vi "ClsSignalIdMakerControl.vi"(11 "SignalIDSettings":T1) -> (3 "Array":i32[](array[numeric]))   [LabVIEW 2015]
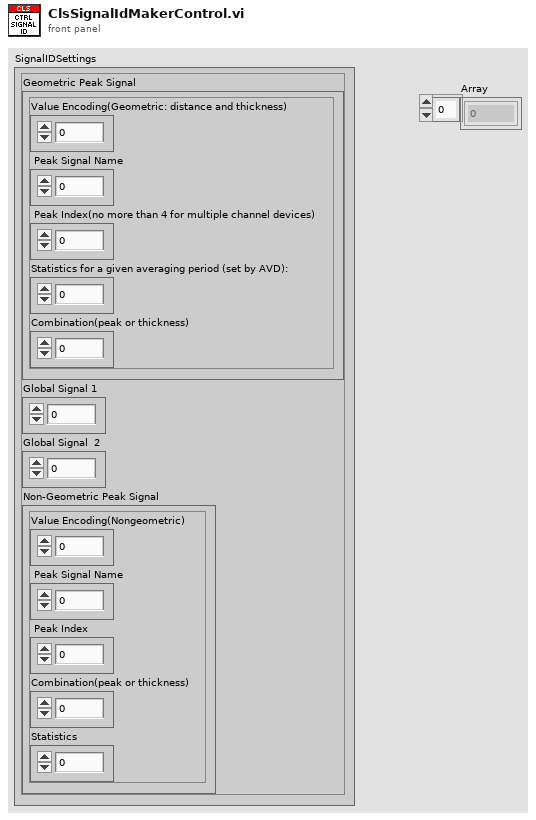
[diagram p1: front panel]
types:
  T1 = cluster{"Geometric Peak Signal":cluster{"Value Encoding(Geometric: distance and thickness) ":i32, " Peak Signal Name":i32, " Peak Index(no more than 4 for multiple channel devices)":i32, "Statistics for a given averaging period (set by AVD):":i32, "Combination(peak or thickness)":i32}, "Global Signal 1":i32, "Global Signal  2":i32, "Non-Geometric Peak Signal":cluster{"Value Encoding(Nongeometric)":i32, " Peak Signal Name":i32, " Peak Index":i32, "Combination(peak or thickness) ":i32, "Statistics":i32}}
  T2 = cluster{"Value Encoding(Nongeometric)":i32, " Peak Signal Name":i32, " Peak Index":i32, "Combination(peak or thickness) ":i32, "Statistics":i32}
  T3 = cluster{"Value Encoding(Geometric: distance and thickness) ":i32, " Peak Signal Name":i32, " Peak Index(no more than 4 for multiple channel devices)":i32, "Statistics for a given averaging period (set by AVD):":i32, "Combination(peak or thickness)":i32}
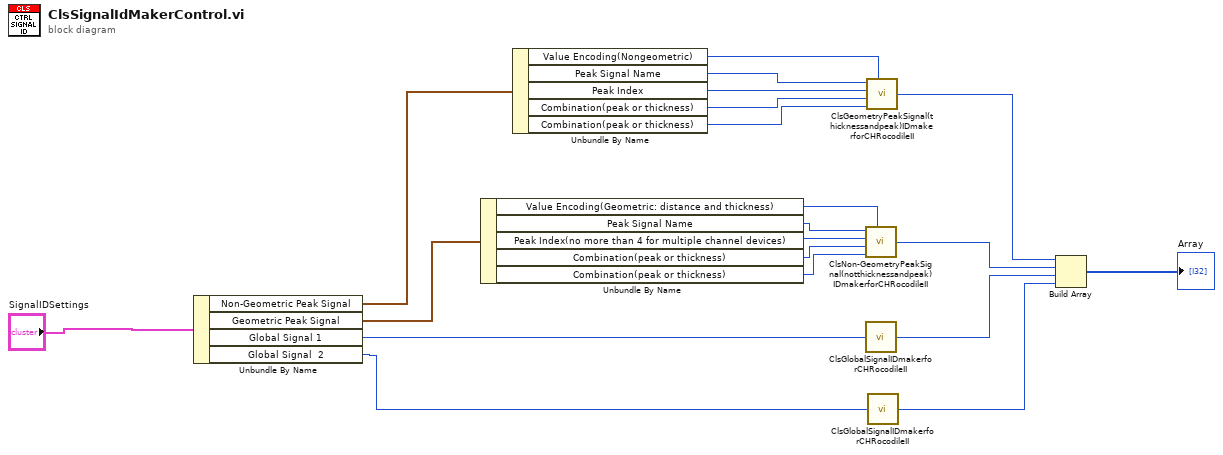
[diagram p0: block diagram]
diagram:
  n1 = Unbundle By Name("SignalIDSettings") -> ("Non-Geometric Peak Signal"=w14:T2, "Geometric Peak Signal"=w15:T3, "Global Signal 1"=w18:i32, "Global Signal  2"=w19:i32)
  n2 = Unbundle By Name(w15) -> ("Value Encoding(Geometric: distance and thickness)"=w7:i32, "Peak Signal Name"=w8:i32, "Peak Index(no more than 4 for multiple channel devices)"=w9:i32, "Combination(peak or thickness)"=w10:i32, "Combination(peak or thickness)"=w11:i32)
  n3 = Unbundle By Name(w14) -> ("Value Encoding(Nongeometric)"=w2:i32, "Peak Signal Name"=w3:i32, "Peak Index"=w4:i32, "Combination(peak or thickness)"=w5:i32, "Combination(peak or thickness)"=w6:i32)
  n4 = call "ClsNon-GeometryPeakSignal(notthicknessandpeak)IDmakerforCHRocodileII.vi"("Peak Signal Name"=w8, "Peak Index"=w9, "Combination(peak or thickness)"=w10, "Statistics"=w11, "Value Encoding(Nongeometric)"=w7) -> ("Non-Geometry Peak Signal ID"=w13:i32)
  n5 = call "ClsGlobalSignalIDmakerforCHRocodileII.vi"("Global Signal Name"=w18) -> ("Global Signal ID"=w16:i32)
  n6 = call "ClsGeometryPeakSignal(thicknessandpeak)IDmakerforCHRocodileII.vi"("Peak Signal Name"=w3, "Peak Index(no more than 4 for multiple channel devices)"=w4, "Combination(peak or thickness)"=w5, "Statistics for a given\naveraging period\n(set by AVD):"=w6, "Value Encoding(Geometric: distance and thickness)"=w2) -> ("Peak Signal ID"=w12:i32)
  n7 = call "ClsGlobalSignalIDmakerforCHRocodileII.vi"("Global Signal Name"=w19) -> ("Global Signal ID"=w17:i32)
  n8 = Build Array(w12, w13, w16, w17) -> (→"Array":i32[])
